vi "Example - Get URL Redirect.vi"() -> ()   [LabVIEW 2019]
uses:
  <vilib>/httpClient/LabVIEWHTTPClient.lvlib
  HTTP Client Extensions.lvlib
panel:
  out "redirect breadcrumb":string[](array[string])
  out "num redirects":i32
  in  "url":string="http://ni.com"
  in  "error in (no error)":errorcluster
  out "error out":errorcluster
  out "redirected?":bool
  out "url out":string
  out "headers":string
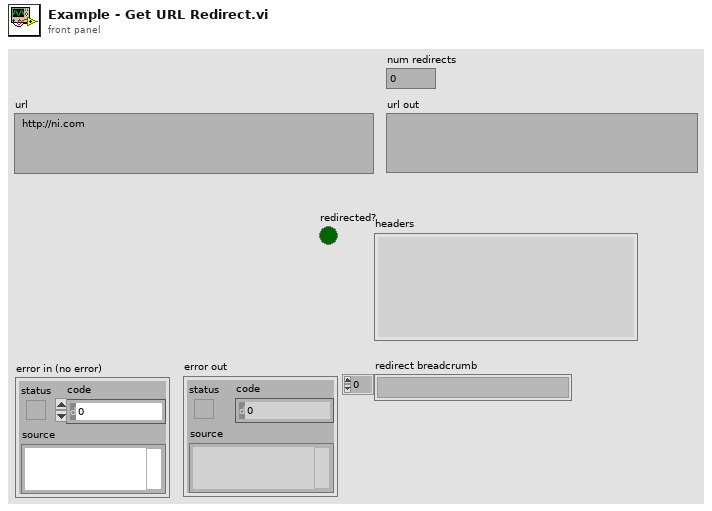
[diagram p1: front panel]
types:
  T1 = typedef "LabVIEWHTTPClient.lvlib/ClientHandle.ctl" = refnum<k1>
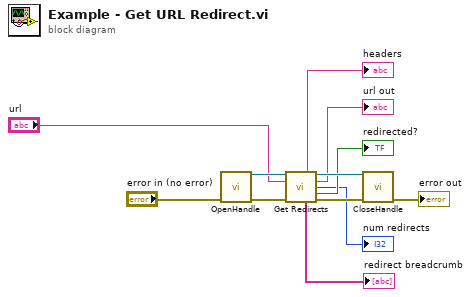
[diagram p0: block diagram]
diagram:
  n1 = call <vilib>:"OpenHandle.vi"("error in (no error)"="error in (no error)") -> ("client handle out"=w10:T1, "error out"=w12:errorcluster)  [unwired: 13 in]
  n2 = call "Get Redirects.vi"("client handle"=w10, "url"="url", "error in (no error)"=w12) -> ("headers"=→"headers":string, "client handle out"=w9:T1, "url out"=→"url out":string, "num redirects"=→"num redirects":i32, "redirected?"=→"redirected?":bool, "redirect breadcrumb"=→"redirect breadcrumb":string[], "error out"=w11:errorcluster)  [unwired: 6 in]
  n3 = call <vilib>:"CloseHandle.vi"("client handle"=w9, "error in (no error)"=w11) -> ("error out"=→"error out":errorcluster)  [unwired: 13 in]
